vi "Scene Settings.vi"(4 "Data Change Event?":bool, 6 "Control Ref Queue":T1, 8 "error in (no error)":errorcluster, 10 "Actual Transform In":T2, 11 "3D Plot.lvclass in":refnum<class "3D Plot.lvclass">) -> (0 "error out":errorcluster, 2 "Actual Transform Out":T2, 3 "3D Plot.lvclass out":refnum<class "3D Plot.lvclass">)   [LabVIEW 2017, in "3D Plot.lvclass"]
uses:
  <vilib>/Math Plots/3D Math Plots/3D Plot/3D Plot/3D Plot.lvclass
  <vilib>/Math Plots/3D Math Plots/3D Plot/3D Plot/Typedef/Actual Transform.ctl
  <vilib>/Math Plots/3D Math Plots/3D Plot/3D Plot/Typedef/Range Clusters.ctl
  <vilib>/Math Plots/3D Math Plots/3D Plot/Action String/3DMathPlot Ctrl Act Queue.ctl
  <vilib>/Math Plots/3D Math Plots/3D Plot/Action String/3DMathPlot Ctrl Act Cluster.ctl
  <vilib>/Math Plots/3D Math Plots/3D Plot/Action String/3DMathPlot State Class.ctl
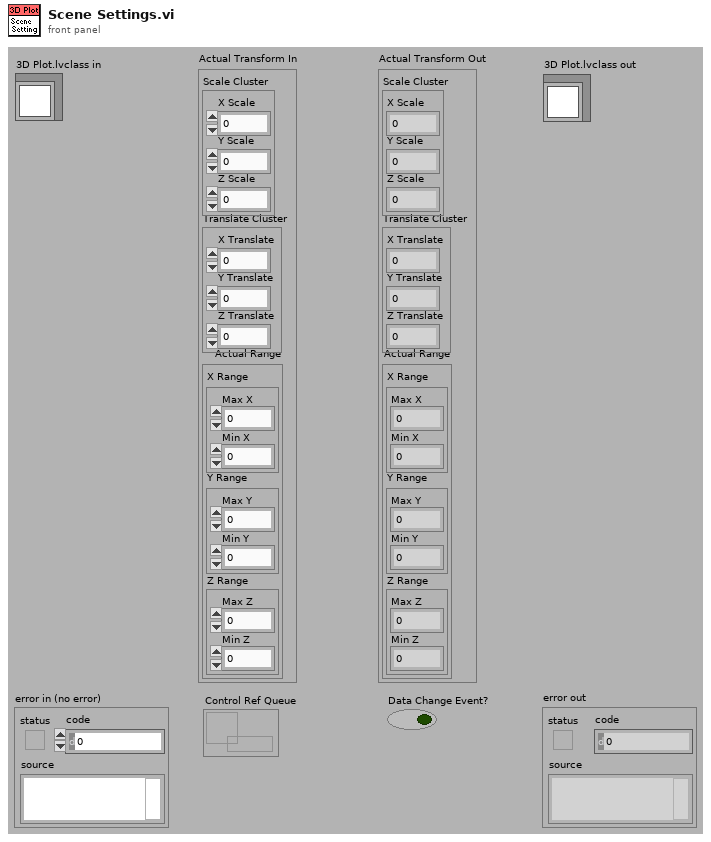
[diagram p1: front panel]
types:
  T1 = typedef "3DMathPlot Ctrl Act Queue.ctl" = refnum<queue>
  T2 = typedef "3D Plot.lvclass/Actual Transform.ctl" = cluster{"Scale Cluster":cluster{"X Scale":sgl, "Y Scale":sgl, "Z Scale":sgl}, "Translate Cluster":cluster{"X Translate":sgl, "Y Translate":sgl, "Z Translate":sgl}, "Actual Range":T3}
  T3 = typedef "3D Plot.lvclass/Range Clusters.ctl" = cluster{"X Range":cluster{"Max X":sgl, "Min X":sgl}, "Y Range":cluster{"Max Y":sgl, "Min Y":sgl}, "Z Range":cluster{"Max Z":sgl, "Min Z":sgl}}
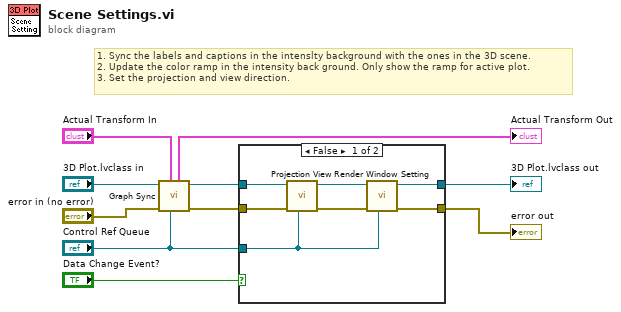
[diagram p0: block diagram]
diagram:
  # "1. Sync the labels and captions in the intenslty background with the ones in the 3D scene.\n2. Update the color ramp in the intensity back ground. Only show the ramp for active plot.\n3. Set the projection and view direction."
  n1 = call <vilib>:"Graph Sync.vi"("Control Ref Queue"="Control Ref Queue", "Actual Transform In"="Actual Transform In", "error in (no error)"="error in (no error)", "3D Plot.lvclass in"="3D Plot.lvclass in") -> ("error out"=w2:errorcluster, "3D Plot.lvclass out"=w3:refnum<class "3D Plot.lvclass">, "Actual Transform Out"=→"Actual Transform Out":T2)  [unwired: 1 in, 4 out]
  n2 = case shown="False" "Data Change Event?" {
    tunnel: [w17 w18] -> w10
    tunnel: [w16 w19] -> w9
    tunnel: "Control Ref Queue" -> [w15 _]
    tunnel: w3 -> [w14 w19]
    tunnel: w2 -> [w13 w18]
    frame False {
      n3 = call <vilib>:"Projection View.vi"("Control Ref Queue"=w15, "error in (no error)"=w13, "3D Plot.lvclass in"=w14) -> ("error out"=w11:errorcluster, "3D Plot.lvclass out"=w12:refnum<class "3D Plot.lvclass">)  [unwired: 1 in, 6 out]
      n4 = call <vilib>:"Render Window Setting.vi"("Control Ref Queue"=w15, "error in (no error)"=w11, "3D Plot.lvclass in"=w12) -> ("error out"=w17:errorcluster, "3D Plot.lvclass out"=w16:refnum<class "3D Plot.lvclass">)  [unwired: 7 out]
    }
    frame True {
    }
  }
  "error out" <- w10
  "3D Plot.lvclass out" <- w9
